vi "Update Channel at Index.vi"(8 "Updated Channel Settings":T2, 9 "Updated Channel Index":i32, 10 "Hardware Configuration from Preview Channel":T1, 11 "Hardware Configuration":T1) -> (1 "Updated Channel Index out":i32, 3 "Hardware Configuration out":T1)   [LabVIEW 2021, in "Settings.lvlib"]
doc: "Replace the channel settings cluster at the index with the new cluster given by 'Updated Channel Settings'."
uses:
  Settings.lvlib
  Acquisition/Channel Settings.ctl
  Acquisition/IO Device.ctl
  Acquisition/Sensor Type.ctl
  Acquisition/Hardware Configuration.ctl
  Interval Timer/Repeat Interval.ctl
  Interval Timer/Interval Length.ctl
  Interval Timer/Interval Token.ctl
  Acquisition/IO Context.ctl
  Acquisition/IO API.ctl
  Acquisition/Acquisition.lvlib
  Interval Timer/Interval Timer.lvlib
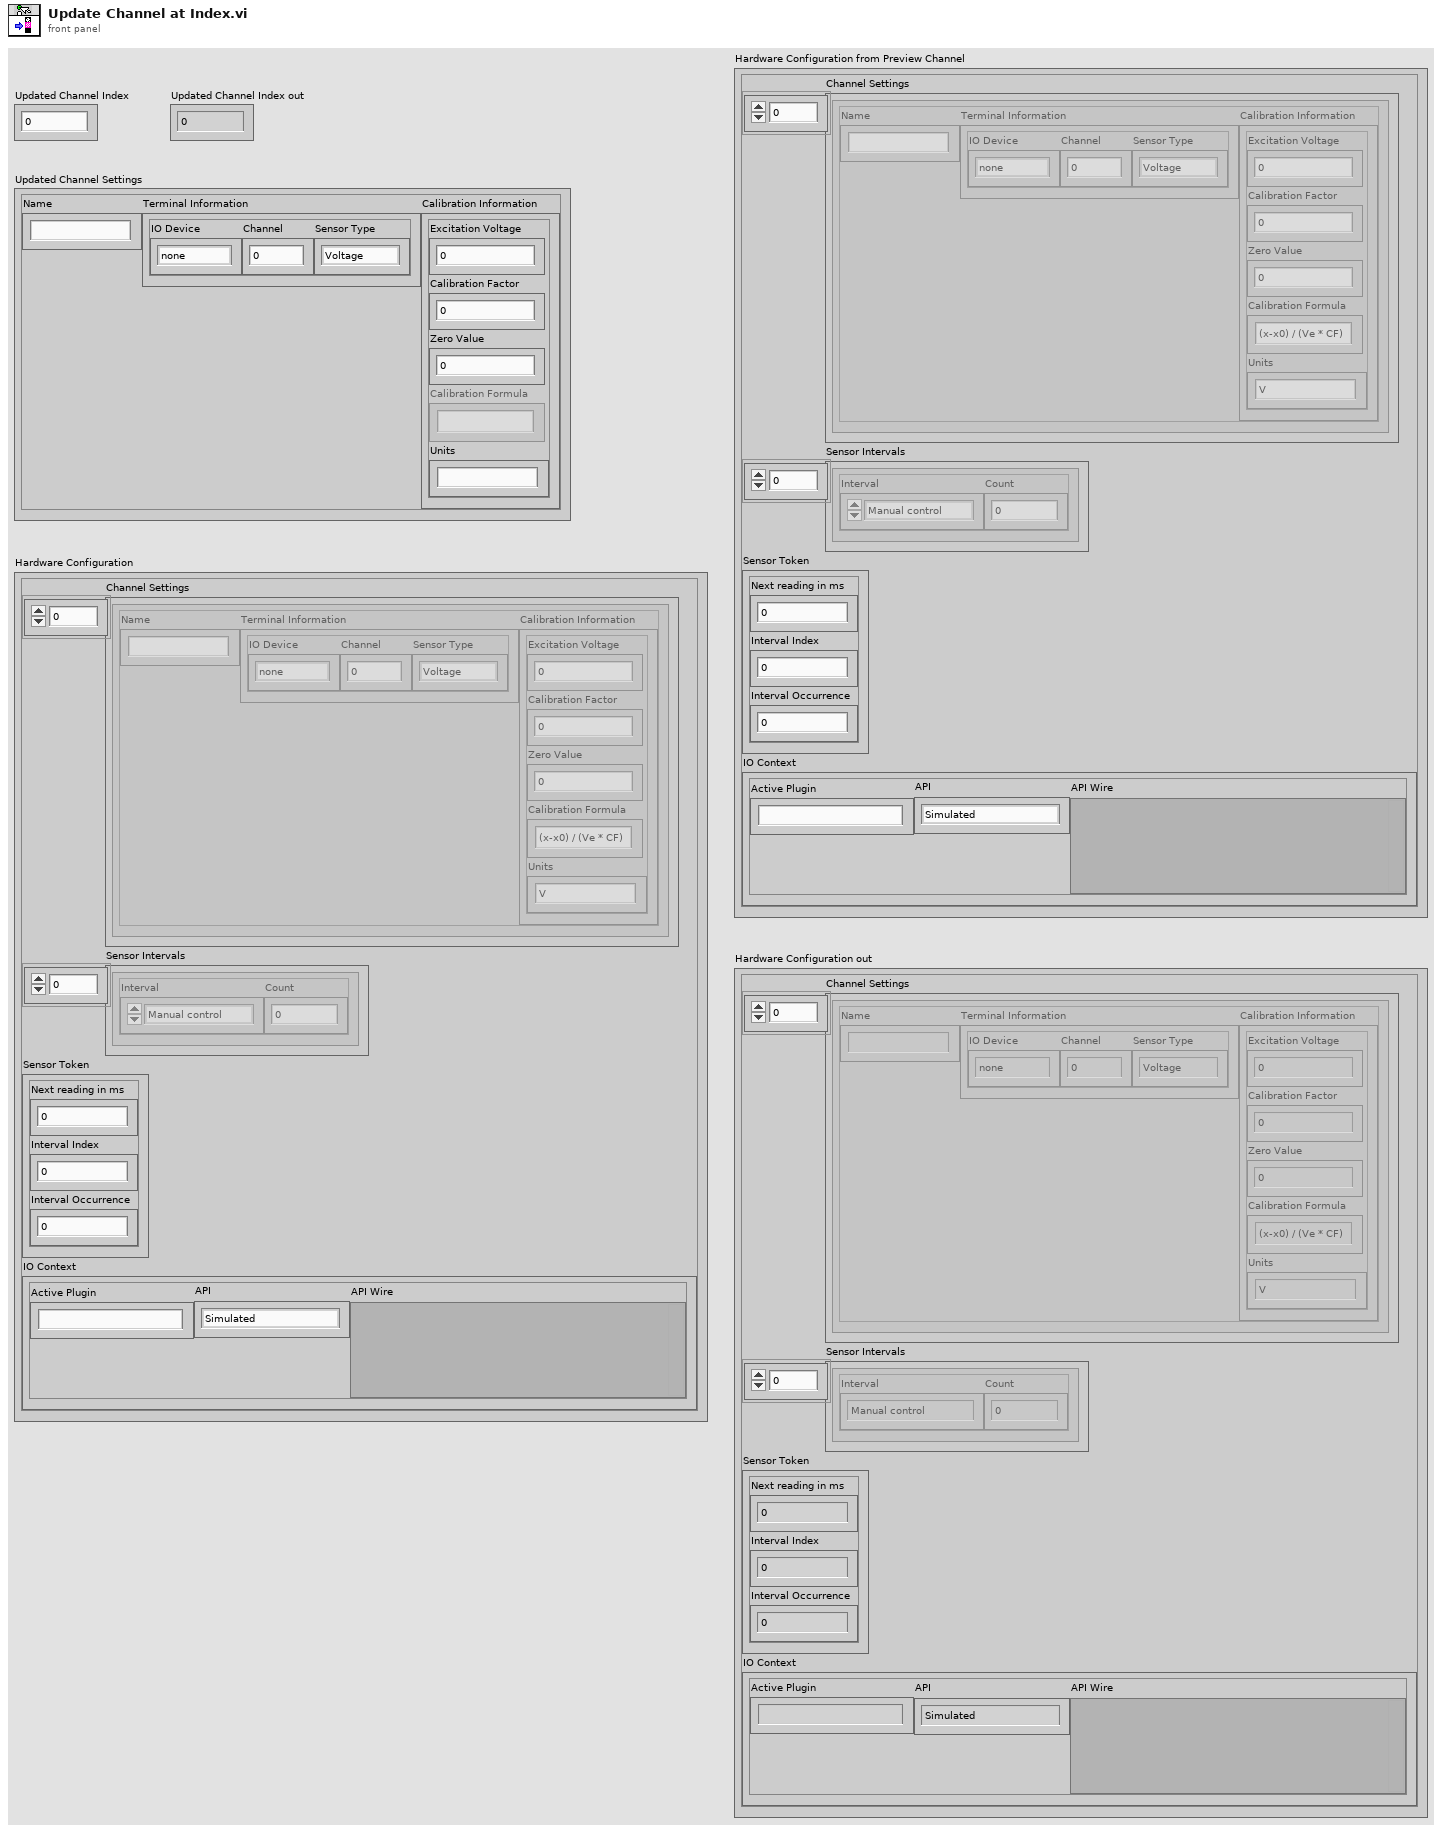
[diagram p1: front panel]
types:
  T1 = typedef "Acquisition.lvlib/Hardware Configuration.ctl" = cluster{"Channel Settings":T2[], "Sensor Intervals":T5[], "Sensor Token":T7, "IO Context":T8}
  T2 = typedef "Acquisition.lvlib/Channel Settings.ctl" = cluster{"Name":string, "Terminal Information":cluster{"IO Device":T3, "Channel":i32, "Sensor Type":T4}, "Calibration Information":cluster{"Excitation Voltage":dbl, "Calibration Factor":dbl, "Zero Value":dbl, "Calibration Formula":string, "Units":string}}
  T3 = typedef "Acquisition.lvlib/IO Device.ctl" = enum16{"none", "9219", "9401"}
  T4 = typedef "Acquisition.lvlib/Sensor Type.ctl" = enum16{"Voltage", "Load", "Pressure", "Encoder"}
  T5 = typedef "Interval Timer.lvlib/Repeat Interval.ctl" = cluster{"Interval":T6, "Count":i32}
  T6 = typedef "Interval Timer.lvlib/Interval Length.ctl" = enum16{"Manual control", "1 second", "10 seconds", "30 seconds", "60 seconds", "600 seconds", "1200 seconds", "3600 seconds"}
  T7 = typedef "Interval Timer.lvlib/Interval Token.ctl" = cluster{"Next reading in ms":u32, "Interval Index":i32, "Interval Occurrence":i32}
  T8 = typedef "Acquisition.lvlib/IO Context.ctl" = cluster{"Active Plugin":string, "API":T9, "API Wire":variant}
  T9 = typedef "Acquisition.lvlib/IO API.ctl" = enum16{"Simulated", "DAQmx"}
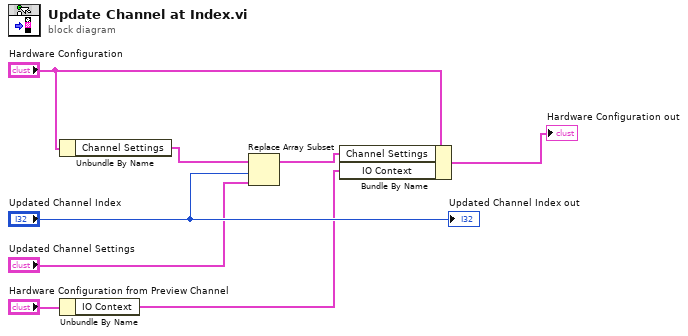
[diagram p0: block diagram]
diagram:
  n1 = Unbundle By Name("Hardware Configuration") -> ("Channel Settings"=w6:T2[])
  n2 = Unbundle By Name("Hardware Configuration from Preview Channel") -> ("IO Context"=w1:T8)
  n3 = Replace Array Subset(array=w6, new element="Updated Channel Settings", index="Updated Channel Index") -> (w3:T2[])
  n4 = Bundle By Name(cluster="Hardware Configuration", "Channel Settings"=w3, "IO Context"=w1) -> (→"Hardware Configuration out":T1)
  "Updated Channel Index out" <- "Updated Channel Index"
